vi "Detect edge.vi"(7 "Filter Type":T2(ring), 8 "error out":errorcluster, 11 "Image In":T1) -> (0 "error out 2":errorcluster, 3 "Image Out":T1)   [LabVIEW 2020]
uses:
  <vilib>/vision/NI_Vision_Development_Module.lvlib
  <vilib>/vision/Image Controls.llb/IMAQ Image.ctl
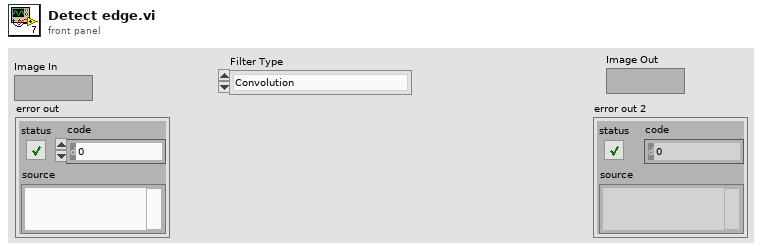
[diagram p1: front panel]
types:
  T1 = typedef "IMAQ Image.ctl" = refnum<image>
  T2 = enum16{"Convolution", "Differentiation", "Gradient", "Prewitt", "Roberts", "Sigma", "Sobel"}
  T3 = enum32{"Differentiation", "Gradient", "Prewitt", "Roberts", "Sigma", "Sobel"}
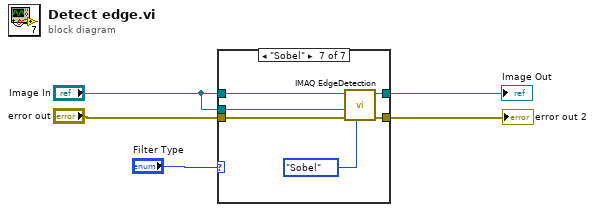
[diagram p0: block diagram]
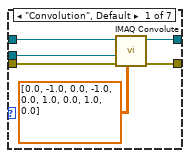
[diagram p2: hidden frame]
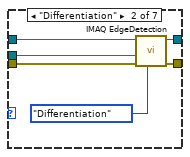
[diagram p3: hidden frame]
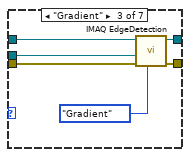
[diagram p4: hidden frame]
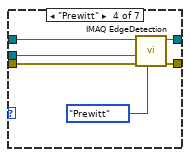
[diagram p5: hidden frame]
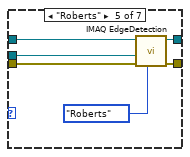
[diagram p6: hidden frame]
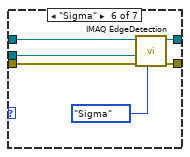
[diagram p7: hidden frame]
diagram:
  n1 = case shown="\"Sobel\"" "Filter Type" {
    tunnel: "Image In" -> [w10 w16 w22 w28 w34 w40 w46]
    tunnel: "error out" -> [w9 w15 w21 w27 w33 w39 w45]
    tunnel: "Image In" -> [w8 w17 w23 w29 w35 w41 w47]
    tunnel: [w7 w12 w18 w24 w30 w36 w42] -> w1
    tunnel: [w6 w13 w19 w25 w31 w37 w43] -> w2
    frame "Convolution", Default {
      n2 = call "IMAQ Convolute"("Kernel"=sgl[][] [[0.0, -1.0, 0.0], [-1.0, 0.0, 1.0], [0.0, 1.0, 0.0]], "error in (no error)"=w9, "Image Dst"=w8, "Image Src"=w10) -> ("error out"=w7:errorcluster, "Image Dst Out"=w6:T1)  [unwired: 6 in]
    }
    frame "Differentiation" {
      n3 = call "IMAQ EdgeDetection"("Method"=T3."Differentiation", "error in (no error)"=w15, "Image Dst"=w17, "Image Src"=w16) -> ("error out"=w12:errorcluster, "Image Dst Out"=w13:T1)  [unwired: 6 in]
    }
    frame "Gradient" {
      n4 = call "IMAQ EdgeDetection"("Method"=T3."Gradient", "error in (no error)"=w21, "Image Dst"=w23, "Image Src"=w22) -> ("error out"=w18:errorcluster, "Image Dst Out"=w19:T1)  [unwired: 6 in]
    }
    frame "Prewitt" {
      n5 = call "IMAQ EdgeDetection"("Method"=T3."Prewitt", "error in (no error)"=w27, "Image Dst"=w29, "Image Src"=w28) -> ("error out"=w24:errorcluster, "Image Dst Out"=w25:T1)  [unwired: 6 in]
    }
    frame "Roberts" {
      n6 = call "IMAQ EdgeDetection"("Method"=T3."Roberts", "error in (no error)"=w33, "Image Dst"=w35, "Image Src"=w34) -> ("error out"=w30:errorcluster, "Image Dst Out"=w31:T1)  [unwired: 6 in]
    }
    frame "Sigma" {
      n7 = call "IMAQ EdgeDetection"("Method"=T3."Sigma", "error in (no error)"=w39, "Image Dst"=w41, "Image Src"=w40) -> ("error out"=w36:errorcluster, "Image Dst Out"=w37:T1)  [unwired: 6 in]
    }
    frame "Sobel" {
      n8 = call "IMAQ EdgeDetection"("Method"=T3."Sobel", "error in (no error)"=w45, "Image Dst"=w47, "Image Src"=w46) -> ("error out"=w42:errorcluster, "Image Dst Out"=w43:T1)  [unwired: 6 in]
    }
  }
  "Image Out" <- w2
  "error out 2" <- w1
